vi "finish_sweep.vi"(8 "error in (no error)":errorcluster, 11 "DataCollectionMG091001IntrinsicImaging in":refnum<class "DataCollectionMG091001IntrinsicImaging.lvclass">) -> (0 "error out":errorcluster, 3 "DataCollectionMG091001IntrinsicImaging out":refnum<class "DataCollectionMG091001IntrinsicImaging.lvclass">)   [LabVIEW 2010, in "DataCollectionMG091001IntrinsicImaging.lvclass"]
uses:
  DataCollectionMG091001IntrinsicImaging.lvclass
  common/classes/ImageCollection/ImageCollection/ImageCollection.lvclass
  DataCollectionMG091001IntrinsicImaging.lvclass/DataCollectionMG091001IntrinsicImaging.ctl
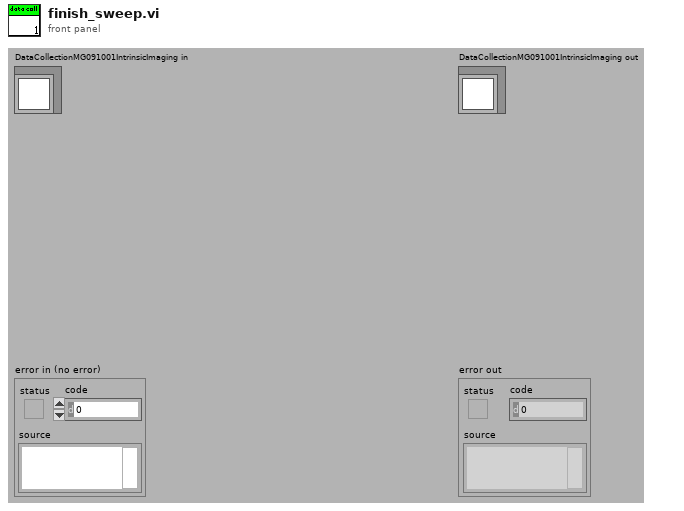
[diagram p1: front panel]
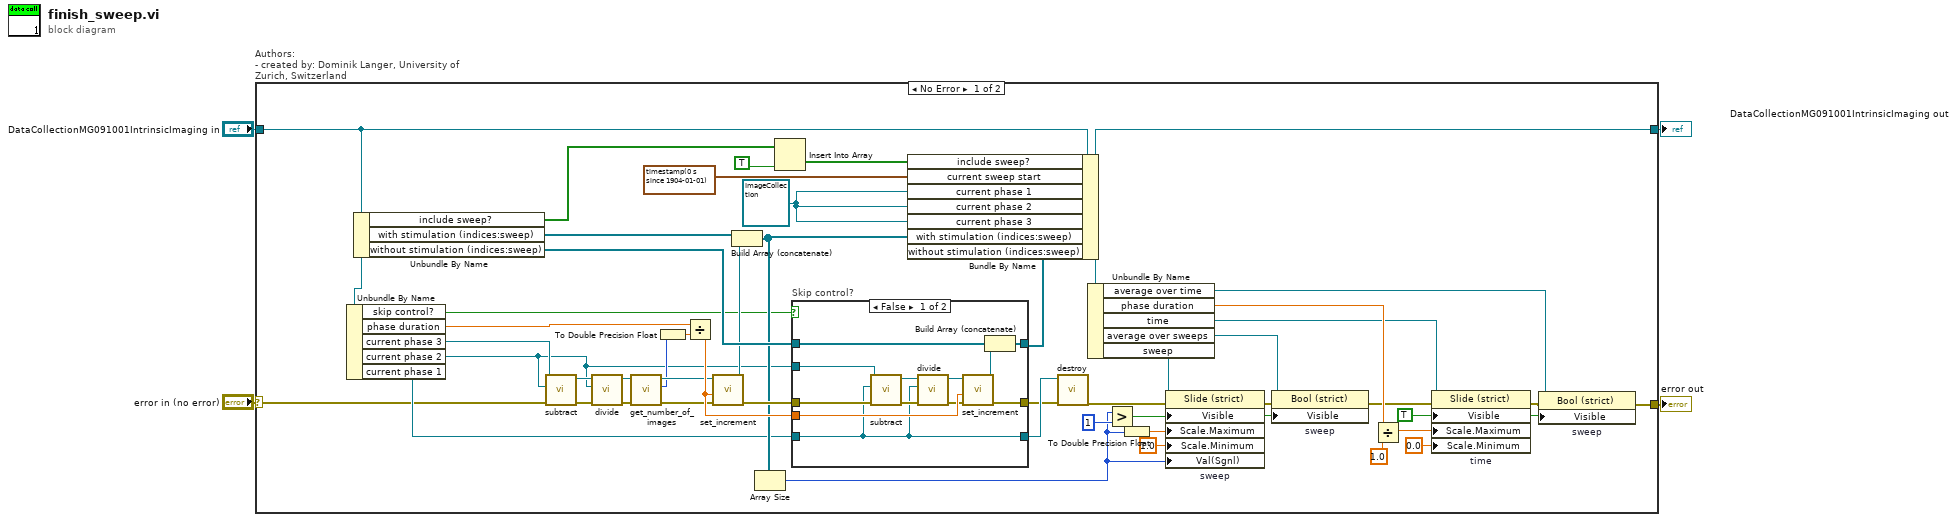
[diagram p0: block diagram]
diagram:
  n1 = case "Authors: \n- created by: Dominik Langer, University of Zurich, Switzerland" shown="No Error" "error in (no error)" {
    selector: "error in (no error)" -> [w8 w70]
    tunnel: [w7 w70] -> w3
    tunnel: [w5 w69] -> w1
    tunnel: "DataCollectionMG091001IntrinsicImaging in" -> [w6 w69]
    frame No Error {
      w21 = TRUE ("Visible")
      w40 = refnum<class "ImageCollection.lvclass"> refnum ("ImageCollection.lvclass")
      n2 = Unbundle By Name(w6) -> ("skip control?"=w16:bool, "phase duration"=w42:dbl[unit], "current phase 3"=w10:refnum<class "ImageCollection.lvclass">, "current phase 2"=w9:refnum<class "ImageCollection.lvclass">, "current phase 1"=w11:refnum<class "ImageCollection.lvclass">)
      n3 = Unbundle By Name(w6) -> ("include sweep?"=w18:bool[], "with stimulation (indices:sweep)"=w46:refnum<class "ImageCollection.lvclass">[], "without stimulation (indices:sweep)"=w53:refnum<class "ImageCollection.lvclass">[])
      n4 = call-dynamic "subtract.vi"("error in (no error)"=w8, "subtrahend"=w9, "ImageCollection in"=w10) -> ("error out"=w15:errorcluster, "ImageCollection out"=w13:refnum<class "ImageCollection.lvclass">)  [unwired: 7 in]
      n5 = call-dynamic "divide.vi"("error in (no error)"=w15, "divisor"=w9, "ImageCollection in"=w13) -> ("error out"=w14:errorcluster, "ImageCollection out"=w12:refnum<class "ImageCollection.lvclass">)  [unwired: 7 in]
      n6 = call-dynamic "get_number_of_images.vi"("error in (no error)"=w14, "ImageCollection in"=w12) -> ("error out"=w45:errorcluster, "size"=w43:i32, "ImageCollection out"=w47:refnum<class "ImageCollection.lvclass">)  [unwired: 7 in]
      n7 = To Double Precision Float(number=w43) -> (double precision float=w44:dbl)
      n8 = Divide(x=w42, y=w44) -> (x/y=w51:dbl[unit])
      n9 = call "set_increment.vi"("error in (no error)"=w45, "time increment"=w51, "ImageCollection in"=w47) -> ("error out"=w49:errorcluster, "ImageCollection out"=w48:refnum<class "ImageCollection.lvclass">)  [unwired: 7 in]
      n10 = Build Array (concatenate)(w46, w48) -> (w36:refnum<class "ImageCollection.lvclass">[])
      n11 = Array Size(array=w36) -> (size(s)=w38:i32)
      n12 = Insert Into Array(array=w18, new element=TRUE ("new element/subarray")) -> (w19:bool[])  [unwired: 1 in]
      n13 = case "Skip control?" shown="False" w16 {
        tunnel: w49 -> [w55 w68]
        tunnel: [w65 w68] -> w50
        tunnel: w11 -> [w54 w67]
        tunnel: w51 -> [w64 _]
        tunnel: w9 -> [w60 _]
        tunnel: [w54 w67] -> w52
        tunnel: w53 -> [w63 w66]
        tunnel: [w61 w66] -> w41
        frame False {
          n14 = call-dynamic "subtract.vi"("error in (no error)"=w55, "subtrahend"=w54, "ImageCollection in"=w60) -> ("error out"=w59:errorcluster, "ImageCollection out"=w57:refnum<class "ImageCollection.lvclass">)  [unwired: 7 in]
          n15 = call-dynamic "divide.vi"("error in (no error)"=w59, "divisor"=w54, "ImageCollection in"=w57) -> ("error out"=w58:errorcluster, "ImageCollection out"=w56:refnum<class "ImageCollection.lvclass">)  [unwired: 7 in]
          n16 = call "set_increment.vi"("error in (no error)"=w58, "time increment"=w64, "ImageCollection in"=w56) -> ("error out"=w65:errorcluster, "ImageCollection out"=w62:refnum<class "ImageCollection.lvclass">)  [unwired: 7 in]
          n17 = Build Array (concatenate)(w63, w62) -> (w61:refnum<class "ImageCollection.lvclass">[])
        }
        frame True {
        }
      }
      n18 = Bundle By Name(cluster=w6, "include sweep?"=w19, "current sweep start"=timestamp(0 s since 1904-01-01) ("y"), "current phase 1"=w40, "current phase 2"=w40, "current phase 3"=w40, "with stimulation (indices:sweep)"=w36, "without stimulation (indices:sweep)"=w41) -> (w5:refnum<class "DataCollectionMG091001IntrinsicImaging.lvclass">)
      n19 = call-dynamic "destroy.vi"("error in (no error)"=w50, "ImageCollection in"=w52) -> ("error out"=w31:errorcluster)  [unwired: 8 in, 1 out]
      n20 = Unbundle By Name(w5) -> ("average over time"=w22:refnum<vi>, "phase duration"=w37:dbl[unit], "time"=w34:refnum<vi>, "average over sweeps"=w26:refnum<vi>, "sweep"=w35:refnum<vi>)
      n21 = Greater?(x=w38, y=1) -> (0:w25:bool)
      n22 = To Double Precision Float(number=w38) -> (double precision float=w33:dbl)
      n23 = property on="sweep" class="Slide (strict)"(reference=w35, error in=w31, "Visible"=w25, "Scale.Maximum"=w33, "Scale.Minimum"=1.0 ("Scale.Range:Minimum"), "Val(Sgnl)"=w38) -> (error out=w27:errorcluster)  [unwired: 1 out]
      n24 = property on="sweep" class="Bool (strict)"(reference=w26, error in=w27, "Visible"=w25) -> (error out=w24:errorcluster)  [unwired: 1 out]
      n25 = Divide(x=w37, y=dbl[unit] 1.0) -> (x/y=w28:dbl)
      n26 = property on="time" class="Slide (strict)"(reference=w34, error in=w24, "Visible"=w21, "Scale.Maximum"=w28, "Scale.Minimum"=0.0 ("Scale.Range:Minimum")) -> (error out=w23:errorcluster)  [unwired: 1 out]
      n27 = property on="sweep" class="Bool (strict)"(reference=w22, error in=w23, "Visible"=w21) -> (error out=w7:errorcluster)  [unwired: 1 out]
    }
    frame Error {
    }
  }
  "error out" <- w3
  "DataCollectionMG091001IntrinsicImaging out" <- w1
